vi "time convector (VLV).vi"(11 "DT_DEC":i32=127) -> (3 "DT_VLV":u8[](array[numeric]) format="%x")   [LabVIEW 2016]
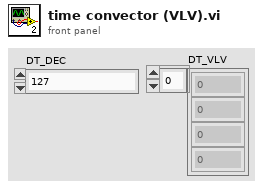
[diagram p1: front panel]
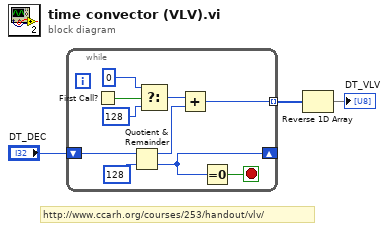
[diagram p0: block diagram]
diagram:
  # "http://www.ccarh.org/courses/253/handout/vlv/"
  n1 = while {
    shift-right: [w10] -> _
    shift-left: "DT_DEC" -> [w12]
    tunnel: [w6] -> w1 mode=indexing
    stop <- w13 stop-if-true
    n2 = First Call?() -> (First Call?: T/F=w9:bool)
    n3 = Quotient & Remainder(x=w12, y=128) -> (x-y*floor(x/y)=w4:i32, floor(x/y)=w10:i32)
    n4 = Select(t=0 ("y"), s=w9, f=128 ("y")) -> (s? t:f=w5:i32)
    n5 = Add(x=w5, y=w4) -> (x+y=w6:i32)
    n6 = Equal To 0?(x=w10) -> (x = 0?=w13:bool)
  }
  n7 = Reverse 1D Array(array=w1) -> (reversed array=→"DT_VLV":i32[])
